vi "Wait-to-Continue.vi"(8 "error in (no error)":errorcluster, 11 "VISA resource name":refnum<visa-resource-name>) -> (0 "error out":errorcluster, 3 "VISA resource name out":refnum<visa-resource-name>)   [LabVIEW 2016, in "Fluke 5XXX Series Multicalibrators.lvlib"]
doc: "This VI Prevents further remote commands from being executed until all previous remote commands have been executed. The *WAI command is useful with any overlapped command, preventing the Calibrator from processing other commands until the overlapped command is processed."
uses:
  Fluke 5XXX Series Multicalibrators.lvlib
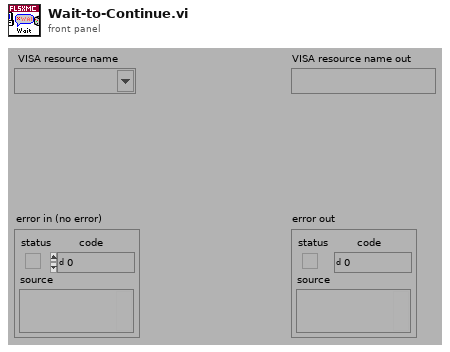
[diagram p1: front panel]
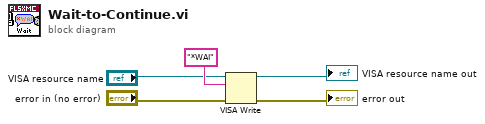
[diagram p0: block diagram]
diagram:
  n1 = VISA Write(VISA resource name="VISA resource name", write buffer="*WAI" ("Reset Command"), error in (no error)="error in (no error)") -> (VISA resource name out=→"VISA resource name out":refnum<visa-resource-name>, error out=→"error out":errorcluster)  [unwired: 1 out]
